vi "U32ArrayToStr(cast).vi"(1 "U32数组":u32[](array[numeric]) format="%.0x") -> (0 "字符串":string)   [LabVIEW 2012]
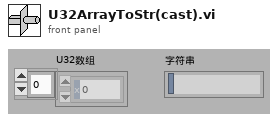
[diagram p1: front panel]
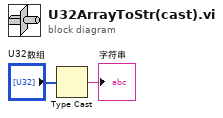
[diagram p0: block diagram]
diagram:
  n1 = Type Cast(x="U32数组") -> (*(type *) &x=→"字符串":string)  [unwired: 1 in]
